vi "nirviSatArithAddEmu(unsigned).vi"(2 "y":u16, 3 "x":u16) -> (0 "overflow":bool, 1 "x+y":u16)   [LabVIEW 2020]
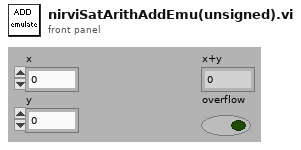
[diagram p1: front panel]
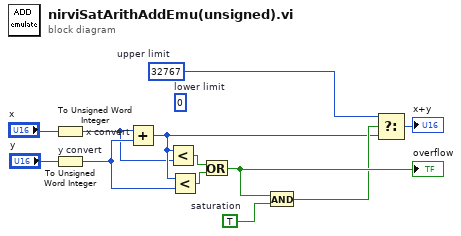
[diagram p0: block diagram]
diagram:
  (unwired) u64 0  # lower limit
  w6 = u16 32767  # upper limit
  w10 = TRUE  # saturation
  n1 = To Unsigned Word Integer "x convert"(number="x") -> (unsigned 16bit integer=w2:u16)
  n2 = To Unsigned Word Integer "y convert"(number="y") -> (unsigned 16bit integer=w4:u16)
  n3 = Add(x=w2, y=w4) -> (x+y=w9:u16)
  n4 = Less?(x=w9, y=w2) -> (x < y?=w8:bool)
  n5 = Less?(x=w9, y=w4) -> (x < y?=w7:bool)
  n6 = Or(x=w8, y=w7) -> (x .or. y?=w12:bool)
  "overflow" <- w12
  n7 = And(x=w12, y=w10) -> (x .and. y?=w11:bool)
  n8 = Select(t=w6, s=w11, f=w9) -> (s? t:f=→"x+y":u16)
